vi "Stop Logging.vi"(0 "reference in":refnum<class "Logger.lvclass">, 11 "Error In":errorcluster) -> (4 "reference out":refnum<class "Logger.lvclass">, 15 "Error Out":errorcluster)   [LabVIEW 2024, in "Logger.lvclass"]
doc: "Closes TDMS file reference in the class properties."
uses:
  Logger.lvclass
panel:
  # "Connector Pane"
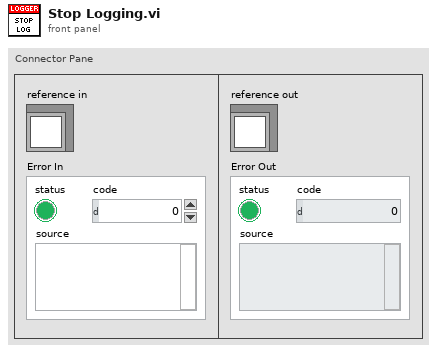
[diagram p1: front panel]
types:
  T1 = typedef "Logger.lvclass/ObjectAttributes.ctl" = cluster{"TDMS File":refnum<k34>, "Channel Names":string[], "Group Name":string}
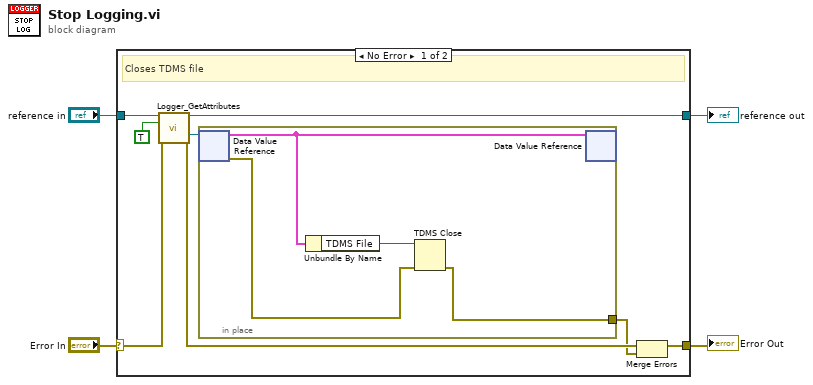
[diagram p0: block diagram]
diagram:
  n1 = case shown="No Error" "Error In" {
    selector: "Error In" -> [w11 w18]
    tunnel: [w9 w18] -> w3
    tunnel: [w10 w17] -> w1
    tunnel: "reference in" -> [w12 w17]
    frame No Error {
      # "Closes TDMS file"
      n2 = call "Logger_GetAttributes.vi"("reference in"=w12, "OnlyGetDvrReference(False)"=TRUE, "Error In"=w11) -> ("reference out"=w10:refnum<class "Logger.lvclass">, "DataRef"=w8:refnum<data-value>, "Error Out"=w7:errorcluster)  [unwired: 9 in, 1 out]
      n3 = in-place {
        in-place-border: [w14] -> w5
        n4 = in-place-dvr #1(w8) -> (w16:T1, w13:errorcluster)
        n5 = Unbundle By Name(w16) -> ("TDMS File"=w15:refnum<k34>)
        n6 = TDMS Close(8:w13, 11:w15) -> (0:w14:errorcluster)  [unwired: 1 out]
        n7 = in-place-dvr #1(w16) -> ()  [unwired: 2 out]
      }
      n8 = Merge Errors(w7, w5) -> (w9:errorcluster)
    }
    frame Error {
    }
  }
  "Error Out" <- w3
  "reference out" <- w1
